vi "Actor Core.vi"(8 "error in":errorcluster caption="entrée d'erreur", 11 "Cooler in":refnum<class "Cooler.lvclass"> caption="Acteur en entrée") -> (0 "error out":errorcluster caption="sortie d'erreur", 3 "Actor out":refnum<class "Actor.lvclass"> caption="Acteur en sortie")   [LabVIEW 2015, in "Cooler.lvlib" / "Cooler.lvclass"]
doc: "(<B>Nom de fichier</B> : Actor Framework.lvlib:Actor.lvclass:Actor Core.vi)\n\nReçoit les messages destinés à l'acteur, y réagit et initialise toute gestion d'erreur susceptible de fermer l'acteur.\n\nLes classes descendantes peuvent redéfinir ce VI pour ajouter des tâches parallèles que l'acteur exécute tout en traitant les messages. Les redéfinitions utilisent le nœud Appeler la méthode parente."
uses:
  Cooler.lvclass
  <vilib>/ActorFramework/Actor/Actor.lvclass
  Dual Controller/Dual Fan/Dual Fan.lvclass
  Water Level/Water Level.lvclass
  Cooler.lvclass/Cooler.ctl
  Level Controller/Level Controller/Level Controller.lvclass
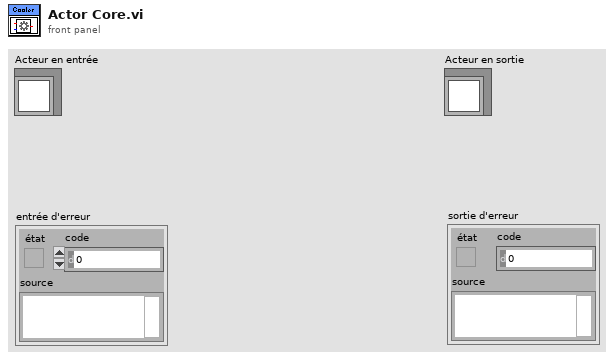
[diagram p1: front panel]
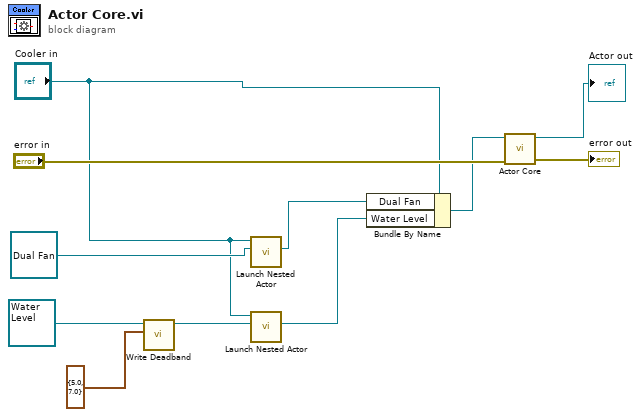
[diagram p0: block diagram]
diagram:
  n1 = call "Write Deadband.vi"("Deadband"=cluster{"LO":dbl, "HI":dbl} {"LO"=5.0, "HI"=7.0}, "Level Controller in"=refnum<class "Water Level.lvclass"> refnum ("Water Level.lvclass")) -> ("Level Controller out"=w5:refnum<class "Water Level.lvclass">)  [unwired: 8 in, 1 out]
  n2 = call <vilib>:"Launch Nested Actor.vi"("Nested Actor"=refnum<class "Dual Fan.lvclass"> refnum ("Dual Fan.lvlib:Dual Fan.lvclass"), "Caller Actor in"="Cooler in") -> ("Nested Actor's Enqueuer"=w3:refnum<class "Message Enqueuer.lvclass">)  [unwired: 7 in, 2 out]
  n3 = call <vilib>:"Launch Nested Actor.vi"("Nested Actor"=w5, "Caller Actor in"="Cooler in") -> ("Nested Actor's Enqueuer"=w2:refnum<class "Message Enqueuer.lvclass">)  [unwired: 7 in, 2 out]
  n4 = Bundle By Name(cluster="Cooler in", "Dual Fan"=w3, "Water Level"=w2) -> (w4:refnum<class "Cooler.lvclass">)
  n5 = call-parent "Actor Core.vi"("error in"="error in", "Timed Loop Controller in"=w4) -> ("error out"=→"error out":errorcluster, "Actor out"=→"Actor out":refnum<class "Actor.lvclass">)  [unwired: 8 in]
